vi "_CH375_Close.vi"(8 "Error In":errorcluster caption="错误输入") -> (0 "Error Out":errorcluster caption="错误输出")   [LabVIEW 2020, in "CH375.lvlib"]
uses:
  CH375.lvlib
  CH375DLL64.dll
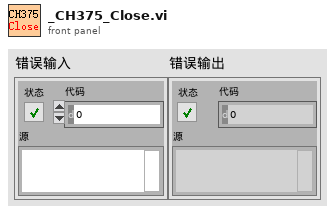
[diagram p1: front panel]
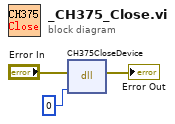
[diagram p0: block diagram]
diagram:
  n1 = dll-call lib="D:/Project NJU/lib/CH375/CH375DLL64.dll" fn="CH375CloseDevice"(error in="Error In", "index"=u32 0) -> (error out=→"Error Out":errorcluster)  [unwired: 3 in, 2 out]
